vi "psk.vi"(0 "Samples per Symbol":i32=8, 1 "PSK System Parameters":T4={"M-PSK (4)"=2, "Differential PSK"=enum."disable", "PSK type"=0} {"PSK type" items=["normal", "shifted", "offset"]}, 2 "System Filter":T8={"TX Filter"=enum."none", "Alpha"=0.5, "Filter Length"=8} {"Alpha" format="%.2f"}, 3 "Symbol Rate, Hz":dbl=100000.0 format="%.2p", 5 "Error In":errorcluster, 6 "Message":T5={"# Guard Bits"=8, "# Sync Bits"=16, "# Message Bits"=2024, "PN sequence order"=9}, 7 "Reset?":bool=TRUE) -> (14 "Measurements":T3={"Frequency Offset (Hz)"=2.406467389382165, "Frequency Drift (Hz)"=16.51402466024529, "Phase Offset (deg)"=-32.81170387840044} {"Phase Offset (deg)" format="%.2f"; "Frequency Drift (Hz)" format="%.2f"; "Frequency Offset (Hz)" format="%.2f"}, 15 "BER":dbl=1.0 format="%.4e", 16 "Accumulated BER":dbl=1.0 format="%.4e", 19 "Error Out":errorcluster={"status"=FALSE, "code"=21848, "source"="my MT PSK Transceiver (One Shot).vi\r\n"})   [LabVIEW 2020]
doc: "This example demonstrates generation and analysis of PSK signals. The example PSK modulates/demodulates a digital message signal and then calculates the bit error rate of the result. Intended as a tool to learn how to program with the Toolkit, this example is similar to another example, MT PSK Transceiver VI, but is less interactive and has simpler underlying LabVIEW code.\n\nThe example generates a digital message with guard, sync, and pn message sequence sections. It modulates the signal and adds white noise to the complex-valued modulated signal samples. The result is demodulated and displayed on constellation (I/Q) plots and digital graphs."
uses:
  <vilib>/measure/mamon.llb/Trigger Detection for 1 Channel.vi
  <vilib>/addons/Modulation/Digital/Demodulation/MT Calculate BER After Trigger (User Pattern).vi
  <vilib>/addons/Modulation/niDMT.lvlib
  <vilib>/measure/NI_MAPro.lvlib
panel:
  in  "FMC Parameters":T1={"IP"="", "Port"=0, "Username"="", "Password"="", "Bandwidth"=18, "Frequency"=2400, "Sample Rate"=30.72, "Buffer Size"=16384}
  out "EVM":T2 {"individual symbol measurements (%)" format="%.2f"; "peak measurement (%)" format="%.2f"; "RMS measurement (%)" format="%.2f"}
  out "tx bit stream ( guard + sync + message )":i8[](array[numeric])
  out "output bit stream":i8[](array[numeric])=[0, 0, 0, 0, 0, 1, 0, 1, 1, 1, 0, 1, 0, 0, 1, 1, 1, 0, 0, 1, 0, 0, 0, 1, 0, 1, 0, 0, 1, 0, 0, 0, 0, 0, 0, 0, 0, 1, 0, 1, 1, 1, 0] caption="bit stream demodulted by labview toolkit"
  out "MER (dB)":dbl format="%.2f"
  out "size(s)":i32
  in  "?":enum32{"Page 1", "Analog Waveform"}(tab)
  out "message bits after demodulated bits":i8[](array[numeric])
  out "sync bits found":bool
  out "message bits found":bool
  out "message bits transmitted":i8[](array[numeric])
  out "Triggered Waveform":dbl[][](graph)
  out "Input Waveform":waveform(dbl)(graph)
  out "Demodulated Waveform":waveform(dbl)(graph)
  in  "Sync Indent, Symbols":i32
  out "BER Trigger\nIndex, Bits":i32
  out "BER Trigger\nFound?":bool
  in  "Tab Control":enum32{"Tx Waveform", "Rx Waveform"}(tab)
  out "Transmitted Constellation":T6(graph)=[{"Decimated Array"=[-4.389014811112454e-17, -4.404483236076944e-17, -5.2475123966416484e-17, 2.6494331318138665e-17, -5.931216780072105e-17, 2.6679952417712547e-17, -4.9412375823447466e-17, -5.0216733921600945e-17, 2.4081257023678226e-17, -5.281542931563527e-17, -4.310125843793555e-17, -4.551433273239599e-17, -4.631869083054947e-17, -4.631869083054947e-17, -4.551433273239599e-17, -4.371999543651515e-17, -5.2629808216061384e-17, 2.6061215419132946e-17, -5.590911430853326e-17, 2.1977551228507588e-17, 1.1273401153080519e-17, 2.197755122850759e-17, -5.652785130711286e-17, 2.5628099520127228e-17, -5.046422872103279e-17, -4.743241742799275e-17, 2.018321393262675e-17, 1.028342195535316e-17, 1.937885583447327e-17, -4.922675472387359e-17], "Decimated Array"=[-0.23842947531470007, -0.2343874450139535, -0.30284933323284813, 0.340743367302347, -0.3599430112308931, 0.34225912866512703, -0.27910240521596225, -0.2856707044546753, 0.32103846958620763, -0.3068913635335947, -0.22756651888144375, -0.24727141659758314, -0.2538397158362963, -0.2538397158362963, -0.24727141659758312, -0.2326190567573769, -0.3053756021708147, 0.3372065907891938, -0.3321540529132606, 0.3038598408080348, 0.21645093555439068, 0.30385984080803474, -0.3372065907891938, 0.3336698142760406, -0.28769171960504863, -0.26293428401297597, 0.28920748096782856, 0.2083668749528976, 0.2826391817291154, -0.2775866438531822]}, {"Decimated Array"=array[480 elements], "Decimated Array"=array[480 elements]}]
  out "Transmitted":T7(graph)={{"1/x"=0.0, 1e-05, [1, 1, 1, 0, 1, 0, 1, 1, 0, 1, 1, 1, 1, 1, 1, 1, 1, 0, 1, 0, 0, 0, 1, 0, 1, 1, 0, 0, 0, 1, 1, 1, 0, 1], 1}, [[0]]}
  out "Received Constellation":T6(graph)=[{"Decimated Array"=[-0.0036950818363619136, 0.019112611831758105, 0.018026314100550018, 0.011658891027980872, 0.04359084781395737, 0.06206914380765105, 0.029702310389105348, 0.07670888353431397, 0.0905867918360375, 0.06207252686340653, 0.024506695990601818, 0.07564480098614051, 0.04377338878992359, 0.021292019212182958, 0.0712462341359347, 0.07918131891296704, 0.06961772578700463, 0.023653818991767276, 0.02989009274416223, 0.020229435777530537, 0.015532330900057902, 0.005173591353259399, 0.04742074049867924, 0.07692049663831156, 0.015376199951295478, 0.06513228218314825, 0.03416798006234203, 0.029133394159845918, 0.053213777831407516, 0.026697258067627527, -0.003994675282759513, -0.0054386722547165684, 0.0011051391041078445, -0.011233603546403369, 0.018414186854903012, 0.024974479460200674, 0.03738224074173192, 0.067614641792115, 0.041168536813839654, 0.054193150807578805, 0.08901109871691629, 0.05614597549146109, 0.036338922528187004], "Decimated Array"=[0.7940860973591571, 0.7889587838492206, 0.7872981517372919, 0.7994208670451515, 0.776651574794085, -1.3362820447241013, 0.8040034250728377, -1.3595195286105504, -1.3189547552723893, -1.3243282178077869, 0.7899324919286101, -1.3490067961499854, 0.8011673602249689, 0.7811848543928405, -1.336855741294819, -1.3167440814864808, -1.3239866386522074, 0.8786559041285253, 0.22994134138912076, -0.4025065174261979, 0.3188116217463296, 0.8383053953283957, 0.7940157900825495, -1.3426559783904723, 0.8020805145535488, -1.3208964432977661, 0.8151621316092003, 0.7857530443584805, -1.3212137682279421, 0.8077411251194435, 0.7836076363886533, 0.7965610412308846, 0.8019367676408321, 0.7933558787025768, 0.7856044652622108, 0.8025249464161269, 0.7779140558433167, -1.3307250825809553, 0.812435327089363, -1.3470539052746473, -1.316401952486522, -1.3168060274197655, 0.8087412291481159]}, {"Decimated Array"=array[688 elements], "Decimated Array"=array[688 elements]}]
  out "Received":T7(graph)={{"1/x"=0.0, 1e-05, [0, 0, 0, 0, 0, 1, 0, 1, 1, 1, 0, 1, 0, 0, 1, 1, 1, 0, 0, 1, 0, 0, 0, 1, 0, 1, 0, 0, 1, 0, 0, 0, 0, 0, 0, 0, 0, 1, 0, 1, 1, 1, 0], 1}, [[0]]}
  in  "Sync Location Uncertainty, Symbols":i32=100
  in  "Expected Sync Location, Symbols":i32
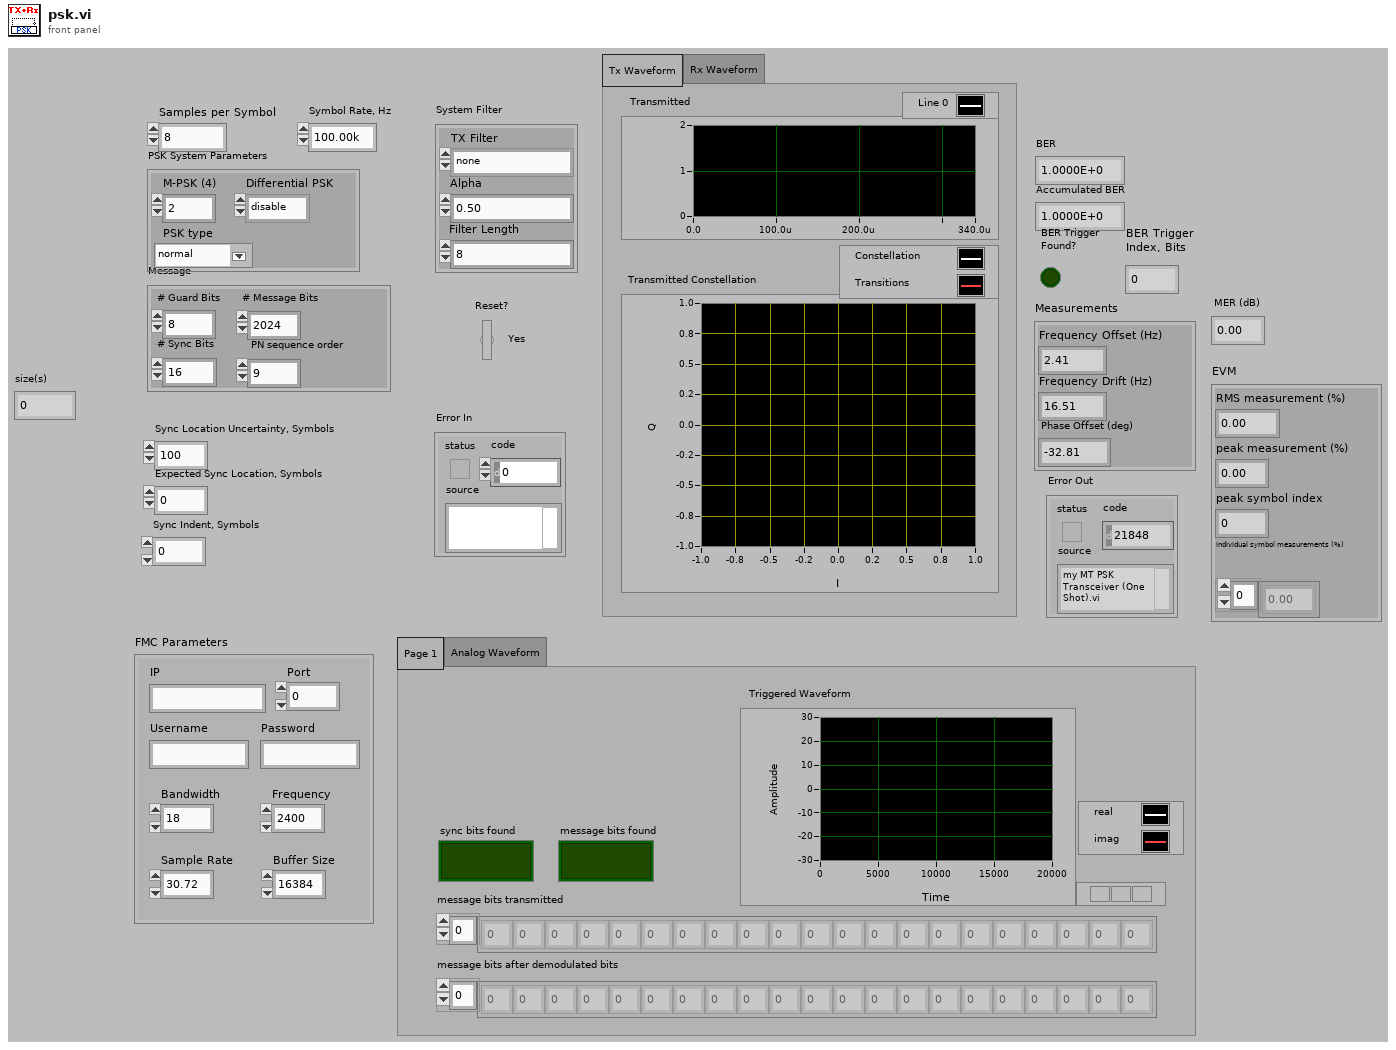
[diagram p1: front panel]
types:
  T1 = cluster{"IP":string, "Port":i32, "Username":string, "Password":string, "Bandwidth":i32, "Frequency":i64, "Sample Rate":dbl, "Buffer Size":i64}
  T2 = cluster{"RMS measurement (%)":dbl, "peak measurement (%)":dbl, "peak symbol index":i32, "individual symbol measurements (%)":dbl[]}
  T3 = cluster{"Frequency Offset (Hz)":dbl, "Frequency Drift (Hz)":dbl, "Phase Offset (deg)":dbl}
  T4 = cluster{"M-PSK (4)":i32, "Differential PSK":enum16{"disable", "enable"}, "PSK type":u16}
  T5 = cluster{"# Guard Bits":i32, "# Sync Bits":i32, "# Message Bits":i32, "PN sequence order":i32}
  T6 = cluster{"Decimated Array":dbl[], "Decimated Array":dbl[]}[]
  T7 = cluster{cluster{"1/x":dbl, dbl, i8[], i32}, i32[][]}
  T8 = cluster{"TX Filter":enum16{"none", "Raised Cosine", "Root Raised Cos", "Gaussian"}, "Alpha":dbl, "Filter Length":i32}
  T9 = cluster{"Expected Sync Location, symbols":i32, "Sync Sequence":cdb[], "Sync Location Uncertainty, symbols":i32, "Sync Indent, symbols":i32}
  T10 = typedef "niDMT.lvlib/PSK System Parameters.ctl" = cluster{"samples per symbol (16)":i32, "symbol map":cdb[], "differential PSK":enum16{"disable", "enable"}, "PSK type":u16}
  T11 = cluster{"Output Bit Stream":i8[], " # bits per symbol":i32, "Sync (Bits)":i8[], "Sync (Symbols)":cdb[], "pulse shaping filter coefficients":dbl[], "matched filter coefficients":dbl[], "PSK system parameters":T10}
  T12 = cluster{"constellation":dbl[], "oversampled data":dbl[]}[]
  T13 = typedef "niAMT.lvlib/Complex Data Waveform.ctl" = cluster{"t0":dbl, "dt":dbl, "Y":cdb[]}
  T14 = cluster{"frequency offset (Hz)":dbl, "frequency drift (Hz)":dbl, "phase offset (deg)":dbl}
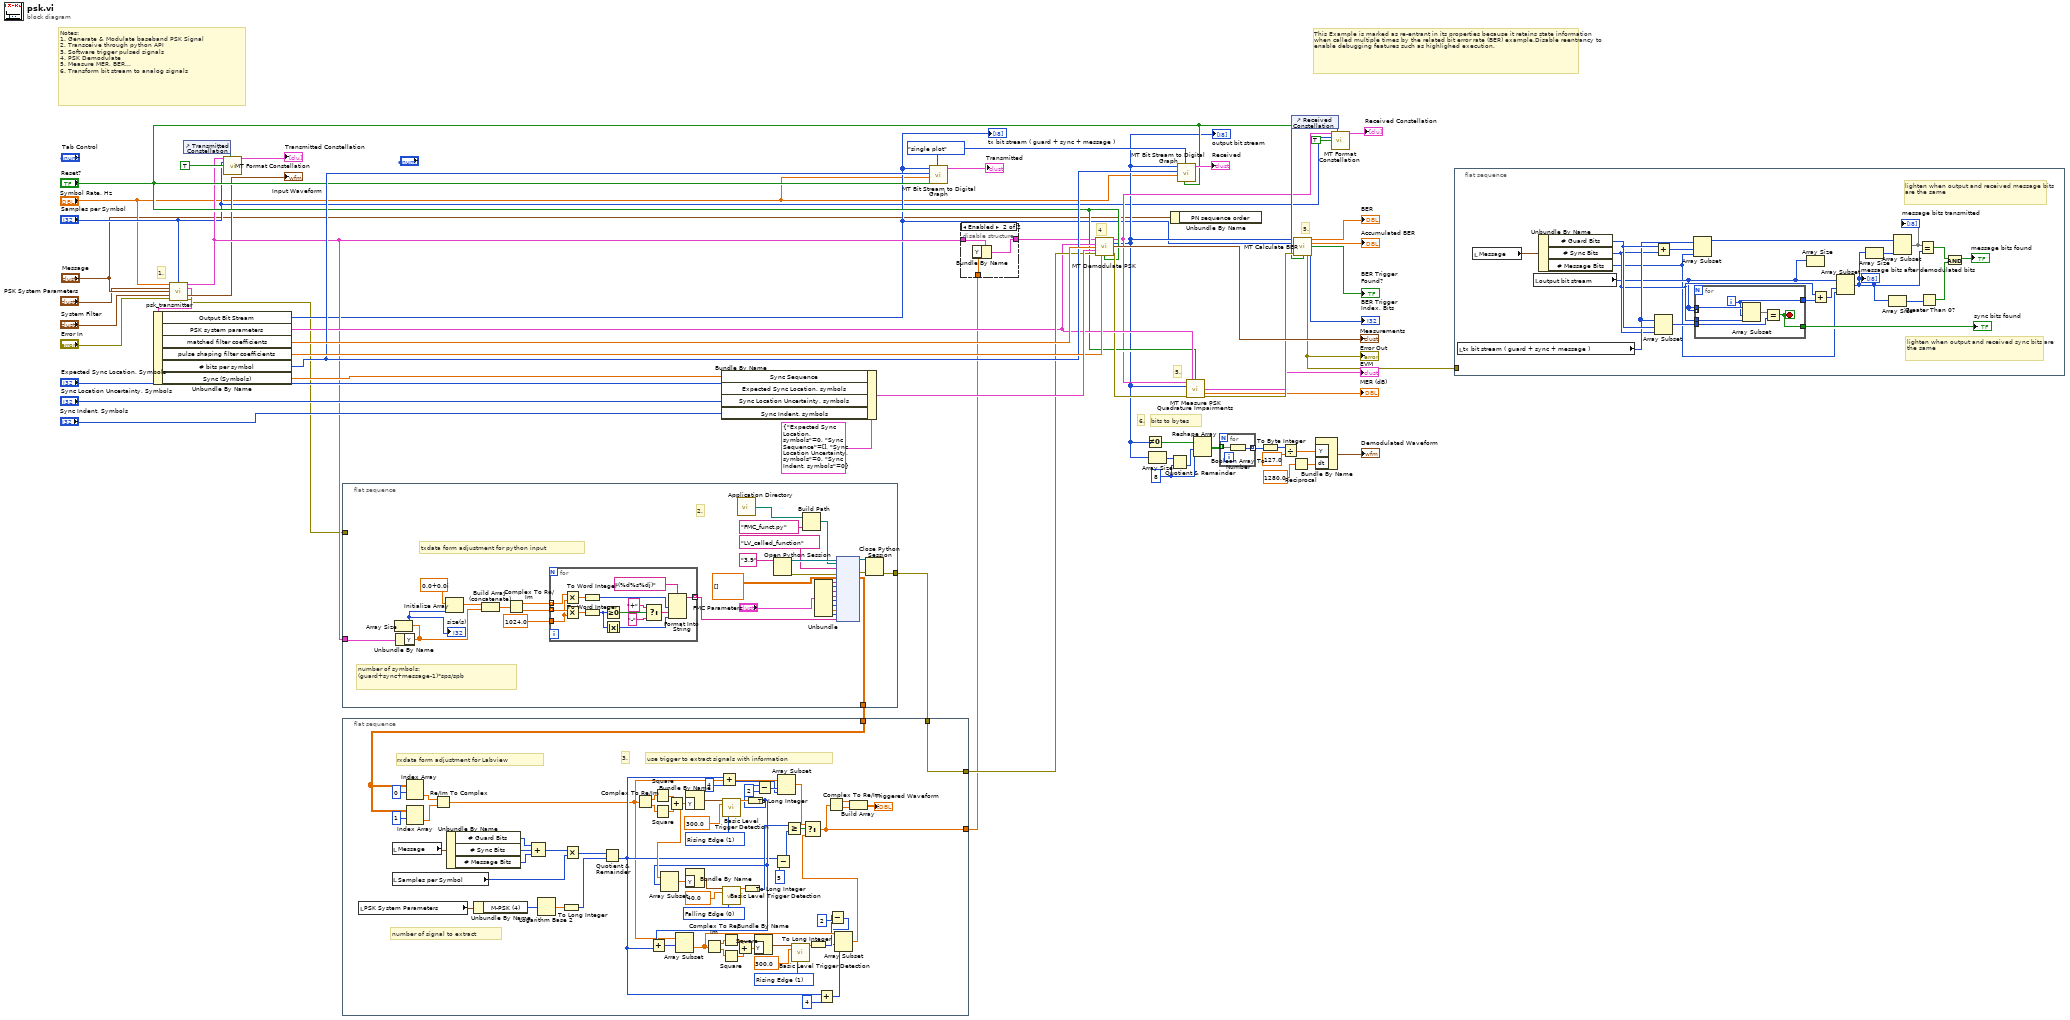
[diagram p0: block diagram]
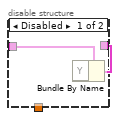
[diagram p2: hidden frame]
diagram:
  w24 = 8
  w49 = enum16{"single plot", "plot per bit"}."single plot" ("Format")
  # "6."
  # "5."
  # "bits to bytes"
  # "This Example is marked as re-entrant in its properties because it retains state information when called multiple times by the related bit error rate (BER) example.Disable reentrancy to enable debugging features such as highlighed execution."
  # "Notes:\n1. Generate & Modulate baseband PSK Signal\n2. Transceive through python API\n3. Software trigger pulsed signals\n4. PSK Demodulate\n5. Measure MER, BER...\n6. Transform bit stream to analog signals"
  # "5."
  # "4"
  # "1."
  n1 = call "psk_transmitter.vi"("Symbol Rate, Hz"="Symbol Rate, Hz", "Samples per Symbol"="Samples per Symbol", "PSK"="PSK System Parameters", "Message"="Message", "System Filter"="System Filter", "error in (no error)"="Error In") -> ("Output Complex Waveform"=w22:cluster{"t0":dbl, "dt":dbl, "Y":cdb[]}, "Signal Description"=w8:T11, "Waveform (analog)"=→"Input Waveform":waveform(dbl), "error out"=w1:errorcluster)  [unwired: 6 in]
  n2 = Unbundle By Name(w8) -> ("Output Bit Stream"=w20:i8[], "PSK system parameters"=w36:T10, "matched filter coefficients"=w53:dbl[], "pulse shaping filter coefficients"=w52:dbl[], "# bits per symbol"=w47:i32, "Sync (Symbols)"=w38:cdb[])
  "tx bit stream ( guard + sync + message )" <- w20
  n3 = control-ref of="Transmitted Constellation"() -> (w44:refnum<vi>)
  n4 = call <vilib>:"MT Format Constellation.vi"("waveform"=w22, "constellation reference"=w44, "samples per symbol"="Samples per Symbol", "autoscale"=TRUE) -> ("constellation graph"=→"Transmitted Constellation":T12)  [unwired: 8 in, 3 out]
  n5 = flat-sequence {
    tunnel: [w91] -> w2
    tunnel: w22 -> [w90]
    tunnel: [w61] -> w3
    tunnel: w1 -> [_]
    frame #0 {
      # "2."
      # "number of symbols:\n(guard+sync+message-1)*sps/spb"
      # "txdata form adjustment for python input"
      n6 = Unbundle By Name(w90) -> ("Y"=w65:cdb[])
      n7 = Array Size(array=w65) -> (size(s)=w63:i32)
      "size(s)" <- w63
      n8 = Initialize Array(cdb 0.0+0.0i, w63) -> (w66:cdb[])
      n9 = Build Array (concatenate)(w66, w65) -> (w67:cdb[])
      n10 = Complex To Re/Im(x + iy=w67) -> (x=w68:dbl[], y=w69:dbl[])
      n11 = for {
        tunnel: w68 -> [w105] mode=indexing
        tunnel: w69 -> [w104] mode=indexing
        tunnel: 1024.0 -> [w103]
        tunnel: [w98] -> w71 mode=indexing
        n12 = Multiply(x=w105, y=w103) -> (x*y=w102:dbl)
        n13 = Multiply(x=w104, y=w103) -> (x*y=w101:dbl)
        n14 = To Word Integer(number=w102) -> (16bit integer=w99:i16)
        n15 = To Word Integer(number=w101) -> (16bit integer=w97:i16)
        n16 = Greater Or Equal To 0?(x=w97) -> (x >= 0?=w96:bool)
        n17 = Absolute Value(x=w97) -> (abs(x)=w92:i16)
        n18 = Select(t="+" ("format string"), s=w96, f="-" ("format string")) -> (s? t:f=w93:string)
        n19 = Format Into String(format string="(%d%s%dj)", w99, w93, w92) -> (resulting string=w98:string)  [unwired: 2 in, 1 out]
      }
      n20 = call <vilib>:"Application Directory.vi"() -> ("Application Directory"=w81:path)
      n21 = Open Python Session(python version="3.9" ("Python version")) -> (session out=w89:refnum<k35>, error out=w88:errorcluster)  [unwired: 2 in]
      n22 = Build Path(base path=w81, name or relative path="FMC_funct.py" ("function name")) -> (appended path=w85:path)
      n23 = Unbundle("FMC Parameters") -> ("IP"=w79:string, "Port"=w78:i32, "Username"=w77:string, "Password"=w76:string, "Bandwidth"=w75:i32, "Frequency"=w74:i64, "Sample Rate"=w73:dbl, "Buffer Size"=w72:i64)
      n24 = node(w89, w85, "LV_called_function" ("function name"), w88, dbl[][] [], w79, w78, w77, w76, w75, w74, w73, w72, w71) -> (w87:refnum<k35>, w86:errorcluster, w61:dbl[][])  [unwired: 9 in, 2 out]
      n25 = Close Python Session(session in=w87, error in=w86) -> (11:w91:errorcluster)
    }
  }
  n26 = flat-sequence {
    tunnel: [w106] -> w37
    tunnel: [w124] -> w30
    tunnel: w3 -> [w112]
    tunnel: w2 -> [w106]
    frame #0 {
      w142 = u16 1 items=["Falling Edge", "Rising Edge"] ("trigger slope")
      w154 = u16 0 items=["Falling Edge", "Rising Edge"] ("trigger slope")
      w162 = u16 1 items=["Falling Edge", "Rising Edge"] ("trigger slope")
      # "rxdata form adjustment for Labview"
      # "3."
      # "number of signal to extract"
      # "use trigger to extract signals with information"
      n27 = local read "PSK System Parameters"() -> (w116:T4)
      n28 = local read "Message"() -> (w167:T5)
      n29 = local read "Samples per Symbol"() -> (w117:i32)
      n30 = Index Array(array=w112, index (row)=0) -> (element=w109:dbl[])  [unwired: 1 in]
      n31 = Index Array(array=w112, index (row)=1) -> (element=w108:dbl[])  [unwired: 1 in]
      n32 = Re/Im To Complex(1:w108, 2:w109) -> (0:w107:cdb[])
      n33 = Unbundle By Name(w167) -> ("# Guard Bits"=w160:i32, "# Sync Bits"=w168:i32, "# Message Bits"=w169:i32)
      n34 = Unbundle By Name(w116) -> ("M-PSK (4)"=w114:i32)
      n35 = Compound Arithmetic op=ADD(w160, w168, w169) -> (w118:i32)
      n36 = Logarithm Base 2(1:w114) -> (0:w115:dbl)
      n37 = To Long Integer(number=w115) -> (32bit integer=w113:i32)
      n38 = Multiply(x=w118, y=w117) -> (x*y=w159:i32)
      n39 = Quotient & Remainder(x=w159, y=w113) -> (floor(x/y)=w119:i32)  [unwired: 1 out]
      n40 = Complex To Re/Im(x + iy=w107) -> (x=w166:dbl[], y=w165:dbl[])
      n41 = Square(x=w166) -> (x^2=w164:dbl[])
      n42 = Square(x=w165) -> (x^2=w163:dbl[])
      n43 = Add(x=w164, y=w163) -> (x+y=w135:dbl[])
      n44 = Bundle By Name("Y"=w135) -> (w152:waveform(dbl))  [unwired: 1 in]
      n45 = Add(x=w119, y=4) -> (x+y=w120:i32)
      n46 = call-poly <vilib>:"Basic Level Trigger Detection.vi"("signal in"=w152, "level"=300.0, "trigger slope"=w162) -> ("trigger location"=w161:dbl)  [unwired: 10 in, 2 out]
      n47 = To Long Integer(number=w161) -> (32bit integer=w130:i32)
      n48 = Add(x=w130, y=w119) -> (x+y=w149:i32)
      n49 = Array Subset(array=w135, index=w130) -> (w136:dbl[])  [unwired: 1 in]
      n50 = Array Subset(array=w107, index=w149) -> (w139:cdb[])  [unwired: 1 in]
      n51 = Bundle By Name("Y"=w136) -> (w137:waveform(dbl))  [unwired: 1 in]
      n52 = Complex To Re/Im(x + iy=w139) -> (x=w145:dbl[], y=w144:dbl[])
      n53 = call-poly <vilib>:"Basic Level Trigger Detection.vi"("signal in"=w137, "level"=40.0, "trigger slope"=w154) -> ("trigger location"=w151:dbl)  [unwired: 10 in, 2 out]
      n54 = Square(x=w145) -> (x^2=w146:dbl[])
      n55 = Square(x=w144) -> (x^2=w143:dbl[])
      n56 = Add(x=w146, y=w143) -> (x+y=w147:dbl[])
      n57 = To Long Integer(number=w151) -> (32bit integer=w132:i32)
      n58 = Bundle By Name("Y"=w147) -> (w148:waveform(dbl))  [unwired: 1 in]
      n59 = Subtract(x=w130, y=2) -> (x-y=w131:i32)
      n60 = Subtract(x=w119, y=5) -> (x-y=w134:i32)
      n61 = Array Subset(array=w107, index=w131, length=w120) -> (w125:cdb[])
      n62 = Greater Or Equal?(x=w132, y=w134) -> (x >= y?=w150:bool)
      n63 = call-poly <vilib>:"Basic Level Trigger Detection.vi"("signal in"=w148, "level"=300.0, "trigger slope"=w142) -> ("trigger location"=w140:dbl)  [unwired: 10 in, 2 out]
      n64 = To Long Integer(number=w140) -> (32bit integer=w127:i32)
      n65 = Add(x=w119, y=4) -> (x+y=w122:i32)
      n66 = Subtract(x=w127, y=2) -> (x-y=w126:i32)
      n67 = Array Subset(array=w139, index=w126, length=w122) -> (w138:cdb[])
      n68 = Select(t=w125, s=w150, f=w138) -> (s? t:f=w124:cdb[])
      n69 = Complex To Re/Im(x + iy=w124) -> (x=w157:dbl[], y=w156:dbl[])
      n70 = Build Array(w157, w156) -> (→"Triggered Waveform":dbl[][])
    }
  }
  n71 = Bundle By Name(cluster=T9 {"Expected Sync Location, symbols"=0, "Sync Sequence"=[], "Sync Location Uncertainty, symbols"=0, "Sync Indent, symbols"=0} ("Synchronization Parameters"), "Sync Sequence"=w38, "Expected Sync Location, symbols"="Expected Sync Location, Symbols", "Sync Location Uncertainty, symbols"="Sync Location Uncertainty, Symbols", "Sync Indent, symbols"="Sync Indent, Symbols") -> (w55:T9)
  n72 = call <vilib>:"MT Bit Stream to Digital Graph.vi"("Reset (F)"="Reset?", "Format"=w49, "Symbol Rate (Hz)"="Symbol Rate, Hz", "bits per symbol"=w47, "Bit Stream"=w20) -> ("Digital Waveform Graph"=→"Transmitted":T7)  [unwired: 6 in]
  n73 = disable-structure shown="Enabled" {
    disable-tunnel: w22 -> [w172 w175]
    disable-tunnel: [w171 w174] -> w31
    disable-tunnel: w30 -> [_ w173]
    frame Disabled {
      n74 = Bundle By Name(cluster=w172) -> (w171:cluster{"t0":dbl, "dt":dbl, "Y":cdb[]}, "Y"=w170:cdb[])
    }
    frame Enabled {
      n75 = Bundle By Name(cluster=w175, "Y"=w173) -> (w174:cluster{"t0":dbl, "dt":dbl, "Y":cdb[]})
    }
  }
  n76 = call <vilib>:"MT Demodulate PSK.vi"("input complex waveform"=w31, "PSK system parameters"=w36, "matched filter coefficients"=w53, "synchronization parameters"=w55, "error in (no error)"=w37, "pulse shaping filter coefficients"=w52, "reset? (T)"="Reset?") -> ("recovered complex waveform"=w29:T13, "output bit stream"=w21:i8[], "measurements"=→"Measurements":T14, "error out"=w35:errorcluster)  [unwired: 3 in, 2 out]
  "output bit stream" <- w21
  n77 = Not Equal To 0?(x=w21) -> (x != 0?=w27:bool[])
  n78 = Array Size(array=w21) -> (size(s)=w26:i32)
  n79 = Unbundle By Name("Message") -> ()  [unwired: 1 out]
  n80 = Quotient & Remainder(x=w26, y=w24) -> (floor(x/y)=w25:i32)  [unwired: 1 out]
  n81 = call <vilib>:"MT Bit Stream to Digital Graph.vi"("Reset (F)"="Reset?", "Format"=w49, "Symbol Rate (Hz)"="Symbol Rate, Hz", "bits per symbol"=w47, "Bit Stream"=w21) -> ("Digital Waveform Graph"=→"Received":T7)  [unwired: 6 in]
  n82 = call <vilib>:"MT Measure PSK Quadrature Impairments.vi"("recovered complex waveform"=w29, "PSK system parameters"=w36, "input bit stream"=w21, "error in (no error)"=w35, "reset? (T)"="Reset?") -> ("EVM"=→"EVM":T2, "modulation error ratio (dB)"=→"MER (dB)":dbl, "error out"=w34:errorcluster)  [unwired: 3 in, 5 out]
  n83 = Reshape Array(w27, w25, w24) -> (w18:bool[][])
  n84 = for {
    tunnel: w18 -> [w177] mode=indexing
    tunnel: [w176] -> w17 mode=indexing
    n85 = Boolean Array To Number(Boolean array=w177) -> (number=w176:u32)
  }
  n86 = To Byte Integer(number=w17) -> (8bit integer=w16:i8[])
  n87 = Divide(x=w16, y=127.0) -> (x/y=w14:dbl[])
  n88 = control-ref of="Received Constellation"() -> (w41:refnum<vi>)
  n89 = Reciprocal(x=1280.0) -> (1/x=w12:dbl)
  n90 = call-poly <vilib>:"MT Calculate BER.vi"("input bit stream"=w21, "reference bit pattern"=w20, "error in (no error)"=w34, "reset? (T)"="Reset?") -> ("BER"=→"BER":dbl, "accumulated BER"=→"Accumulated BER":dbl, "trigger found?"=→"BER Trigger\nFound?":bool, "trigger found index (bits)"=→"BER Trigger\nIndex, Bits":u32, "error out"=w32:errorcluster)  [unwired: 7 in]
  "Error Out" <- w32
  n91 = Bundle By Name("Y"=w14, "dt"=w12) -> (→"Demodulated Waveform":waveform(dbl))  [unwired: 1 in]
  n92 = call <vilib>:"MT Format Constellation.vi"("waveform"=w29, "constellation reference"=w41, "samples per symbol"="Samples per Symbol", "autoscale"=TRUE) -> ("constellation graph"=→"Received Constellation":T12)  [unwired: 8 in, 3 out]
  n93 = flat-sequence {
    tunnel: w32 -> [_]
    frame #0 {
      # "lighten when output and received message bits are the same"
      # "lighten when output and received sync bits are the same"
      n94 = local read "tx bit stream ( guard + sync + message )"() -> (w189:i8[])
      n95 = local read "Message"() -> (w191:T5)
      n96 = local read "output bit stream"() -> (w181:i8[])
      n97 = Unbundle By Name(w191) -> ("# Guard Bits"=w190:i32, "# Sync Bits"=w183:i32, "# Message Bits"=w178:i32)
      n98 = Array Subset(array=w189, index=w190, length=w183) -> (w196:i8[])
      n99 = Add(x=w190, y=w183) -> (x+y=w193:i32)
      n100 = Array Subset(array=w189, index=w193, length=w178) -> (w192:i8[])
      n101 = for {
        tunnel: w181 -> [_] mode=indexing
        tunnel: w181 -> [w202]
        tunnel: w183 -> [w201]
        tunnel: w196 -> [w199]
        tunnel: [w198] -> w195
        tunnel: [w197] -> w185
        i -> [w198]
        stop <- w197 stop-if-true
        n102 = Array Subset(array=w202, index=w198, length=w201) -> (w200:i8[])
        n103 = Equal?(x=w200, y=w199) -> (x = y?=w197:bool)
      }
      "sync bits found" <- w185
      n104 = Array Size(array=w181) -> ()  [unwired: 1 out]
      n105 = Add(x=w183, y=w195) -> (x+y=w194:i32)
      n106 = Array Subset(array=w181, index=w194, length=w178) -> (w180:i8[])
      "message bits after demodulated bits" <- w180
      n107 = Array Size(array=w180) -> (size(s)=w182:i32)
      n108 = Array Size(array=w180) -> (size(s)=w188:i32)
      n109 = Array Subset(array=w192, length=w182) -> (w179:i8[])  [unwired: 1 in]
      "message bits transmitted" <- w179
      n110 = Equal?(x=w179, y=w180) -> (x = y?=w187:bool)
      n111 = Greater Than 0?(x=w188) -> (x > 0?=w186:bool)
      n112 = And(x=w187, y=w186) -> (x .and. y?=→"message bits found":bool)
    }
  }
